vi "LOOP ARM POSITION.vi"(1 "LEFT-RIGHT":string="LEFT", 5 "error in (no error)":errorcluster, 7 "PID Constants ARM":T2={"P Gain"=0.0, "I Gain"=0.0, "D Gain"=0.0, "F Gain"=0.0, "I Zone"=0.0, "Min Output"=-1.0, "Max Output"=1.0} {"Max Output" min=-1.0 max=1.0 step=0.01; "Min Output" min=-1.0 max=1.0 step=0.01; "I Zone" step=0.01; "F Gain" step=0.01; "D Gain" step=0.01; "I Gain" step=0.01; "P Gain" min=0.0 step=0.01}) -> (19 "error out":errorcluster)   [LabVIEW 2020]
uses:
  <vilib>/Rock Robotics/WPI/MotorControl/WPI_MotorControlDeviceRef.ctl
  <vilib>/Rock Robotics/WPI/MotorControl/WPI_MotorControlType.ctl
  <vilib>/Rock Robotics/SystemInterfaces/DIO/FPGA_DIOPWMChannel.ctl
  <vilib>/Rock Robotics/WPI/PWM/WPI_PWMDeadband.ctl
  <vilib>/Rock Robotics/SystemInterfaces/DIO/FPGA_DIOChannel.ctl
  <vilib>/Rock Robotics/WPI/ThirdParty/REV Robotics/REVLib/Typedef/Spark MAX Control Type.ctl
  <vilib>/Rock Robotics/WPI/ThirdParty/REV Robotics/REVLib/Typedef/Spark MAX Limit Direction.ctl
  Robot Global Data.vi
  <vilib>/Rock Robotics/Network Tables/NT Read Number.vi
  <vilib>/Rock Robotics/Network Tables/NT Write Number.vi
panel:
  in  "INPUT STROKE":dbl(slide) min=0.0 max=23.5 scale=0.0..23.5
  in  "INPUT ARM":dbl(slide) min=-3.5 max=4.5 scale=-3.5..4.5
  in  "TESTING?":bool
  out "REV Limit":T1
  out "FWD Limit":T1
  in  "PID Constants Climber":T2={"P Gain"=0.0, "I Gain"=0.0, "D Gain"=0.0, "F Gain"=0.0, "I Zone"=0.0, "Min Output"=-1.0, "Max Output"=1.0} {"Max Output" min=-1.0 max=1.0 step=0.01; "Min Output" min=-1.0 max=1.0 step=0.01; "I Zone" step=0.01; "F Gain" step=0.01; "D Gain" step=0.01; "I Gain" step=0.01; "P Gain" min=0.0 step=0.01}
  out "Position 2":dbl
  out "Output 2":dbl
  out "PID Chart STROKE":T3(graph)
  in  "NT arm string":string="ARM"
  in  "nt set pos string":string="/setPOS"
  out "MotorControlDevRef out":T4={"DeviceStatus"={"status"=FALSE, "code"=0, "source"=""}, "Type"=enum."PWM", "PWM"={"PWM Channel"=enum."Invalid", "DeadBand"={"Name"="", "maxPositivePwm"=0, "minPositivePwm"=0, "centerPwm"=0, "maxNegativePwm"=0, "minNegativePwm"=0, "angularRange"=0}}, "CAN"={"Device Number"=0, "SetOutput VI Ref"=variant, "GetOutput VI Ref"=variant, "Enable VI Ref"=variant, "Disable VI Ref"=variant, "Data"=variant}, "Invert"=FALSE, "DIO PWM"={"PWM \"Enable\" Channel"=enum."Invalid", "DIOChannel"=enum."Invalid", "PWM Rate"=0.0}}
  out "Position":dbl
  out "Output":dbl
  in  "ARM devref in":T4={"DeviceStatus"={"status"=FALSE, "code"=0, "source"=""}, "Type"=enum."PWM", "PWM"={"PWM Channel"=enum."Invalid", "DeadBand"={"Name"="", "maxPositivePwm"=0, "minPositivePwm"=0, "centerPwm"=0, "maxNegativePwm"=0, "minNegativePwm"=0, "angularRange"=0}}, "CAN"={"Device Number"=0, "SetOutput VI Ref"=variant, "GetOutput VI Ref"=variant, "Enable VI Ref"=variant, "Disable VI Ref"=variant, "Data"=variant}, "Invert"=FALSE, "DIO PWM"={"PWM \"Enable\" Channel"=enum."Invalid", "DIOChannel"=enum."Invalid", "PWM Rate"=0.0}}
  out "PID Chart ANGLE":T3(graph)
  # "EXECUTION to SHARED RE-ENTRANT"
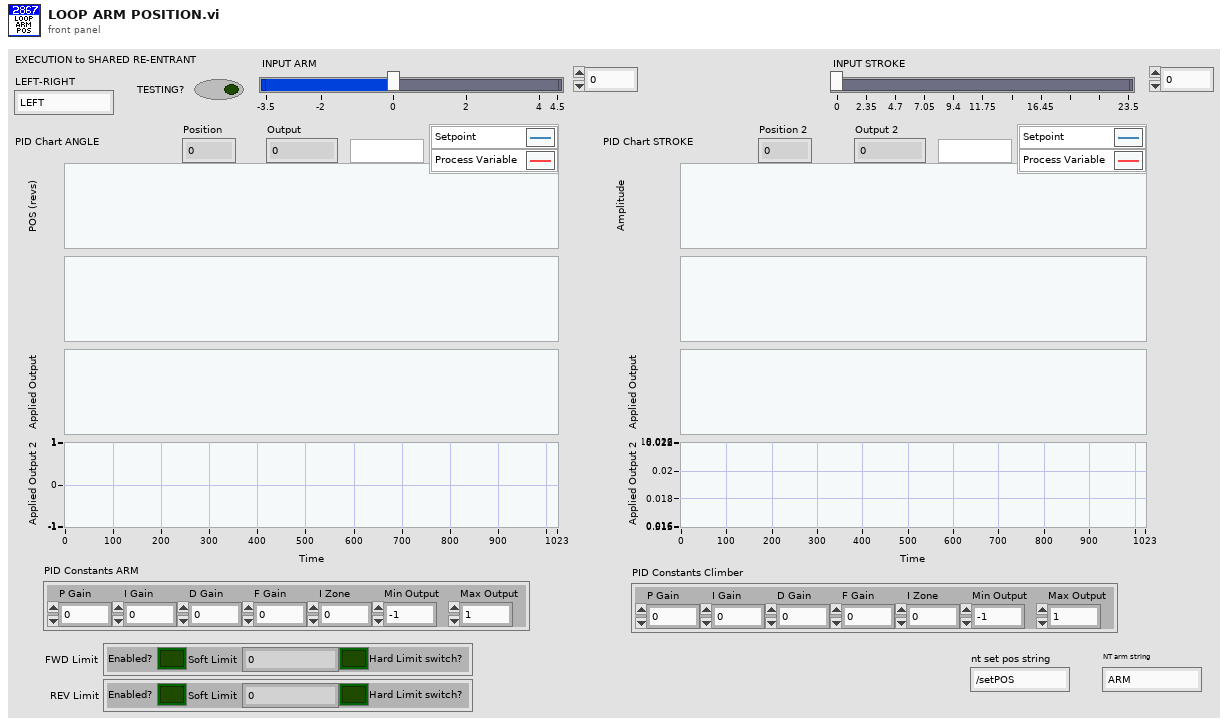
[diagram p1: front panel]
types:
  T1 = cluster{"Enabled?":bool, "Soft Limit":dbl, "Hard Limit switch?":bool}
  T2 = cluster{"P Gain":dbl, "I Gain":dbl, "D Gain":dbl, "F Gain":dbl, "I Zone":dbl, "Min Output":dbl, "Max Output":dbl}
  T3 = cluster{"Sensor Position":dbl, "Sensor Position":dbl, "Setpoint":dbl, "Applied Output":dbl}
  T4 = typedef "WPI_MotorControlDeviceRef.ctl" = cluster{"DeviceStatus":errorcluster, "Type":T5, "PWM":cluster{"PWM Channel":T6, "DeadBand":T7}, "CAN":cluster{"Device Number":u8, "SetOutput VI Ref":variant, "GetOutput VI Ref":variant, "Enable VI Ref":variant, "Disable VI Ref":variant, "Data":variant}, "Invert":bool, "DIO PWM":cluster{"PWM \"Enable\" Channel":T6, "DIOChannel":T8, "PWM Rate":dbl}}
  T5 = typedef "WPI_MotorControlType.ctl" = enum16{"PWM", "CAN", "DIO PWM"}
  T6 = typedef "FPGA_DIOPWMChannel.ctl" = enum8{"PWM 0", "PWM 1", "PWM 2", "PWM 3", "PWM 4", "PWM 5", "PWM 6", "PWM 7", "PWM 8", "PWM 9", "PWM MXP 0", "PWM MXP 1", "PWM MXP 2", "PWM MXP 3", "PWM MXP 4", "PWM MXP 5", "PWM MXP 6", "PWM MXP 7", "PWM MXP 8", "PWM MXP 9", "Invalid"}
  T7 = typedef "WPI_PWMDeadband.ctl" = cluster{"Name":string, "maxPositivePwm":i32, "minPositivePwm":i32, "centerPwm":i32, "maxNegativePwm":i32, "minNegativePwm":i32, "angularRange":u16}
  T8 = typedef "FPGA_DIOChannel.ctl" = enum8{"DIO 0", "DIO 1", "DIO 2", "DIO 3", "DIO 4", "DIO 5", "DIO 6", "DIO 7", "DIO 8", "DIO 9", "DIO MXP 0", "DIO MXP 1", "DIO MXP 2", "DIO MXP 3", "DIO MXP 4", "DIO MXP 5", "DIO MXP 6", "DIO MXP 7", "DIO MXP 8", "DIO MXP 9", "DIO MXP 10", "DIO MXP 11", "DIO MXP 12", "DIO MXP 13", "DIO MXP 14", "DIO MXP 15", "SPI Port CS1", "SPI Port CS2", "SPI Port CS3", "SPI Port MISO", "SPI Port MOSI", "Invalid"}
  T9 = cluster{"MIN":dbl, "MAX":dbl, "convert climber inches to tics":dbl}
  T10 = cluster{"MIN":dbl, "MAX":dbl, "convert arm inches to revs":dbl}
  T11 = typedef "Spark MAX Control Type.ctl" = enum16{"Percent VBus", "Voltage", "Velocity", "Position", "Smart Motion", "Current", "Smart Velocity"}
  T12 = typedef "Spark MAX Limit Direction.ctl" = enum16{"Forward Limit", "Reverse Limit"}
  T13 = cluster{"P Gain":bool, "I Gain":bool, "D Gain":bool, "F Gain":bool, "I Zone":bool, "Min Output":bool, "Max Output":bool}
  T14 = typedef "Spark MAX Status 2 Frame.ctl" = cluster{"Sensor Position":dbl, "IAccum":dbl, "Timestamp":u32}
  T15 = typedef "Spark MAX Status 0 Frame.ctl" = cluster{"Applied Output":dbl, "Faults":T16, "Sticky Faults":T16, "Rsvd":u8, "Status 0 Flags":T17, "Timestamp":u32}
  T16 = typedef "Spark MAX Faults.ctl" = cluster{"Hard Limit Rev":bool, "Hard Limit Fwd":bool, "Soft Limit Fwd":bool, "Soft Limit Rev":bool, "Other Fault":bool, "DRV Fault":bool, "Has Reset?":bool, "CAN RX":bool, "CAN TX":bool, "EEPROM CRC":bool, "Stall":bool, "Sensor Fault":bool, "Motor Type Fault":bool, "IWDT Reset":bool, "Over Current":bool, "Brownout":bool}
  T17 = typedef "Spark MAX Status 0 Flags.ctl" = cluster{"Invert/Brake":bool, "Is Follower":bool}
  T18 = cluster{"Sensor Position":dbl, "Sensor Position":dbl, dbl, "Applied Output":dbl}
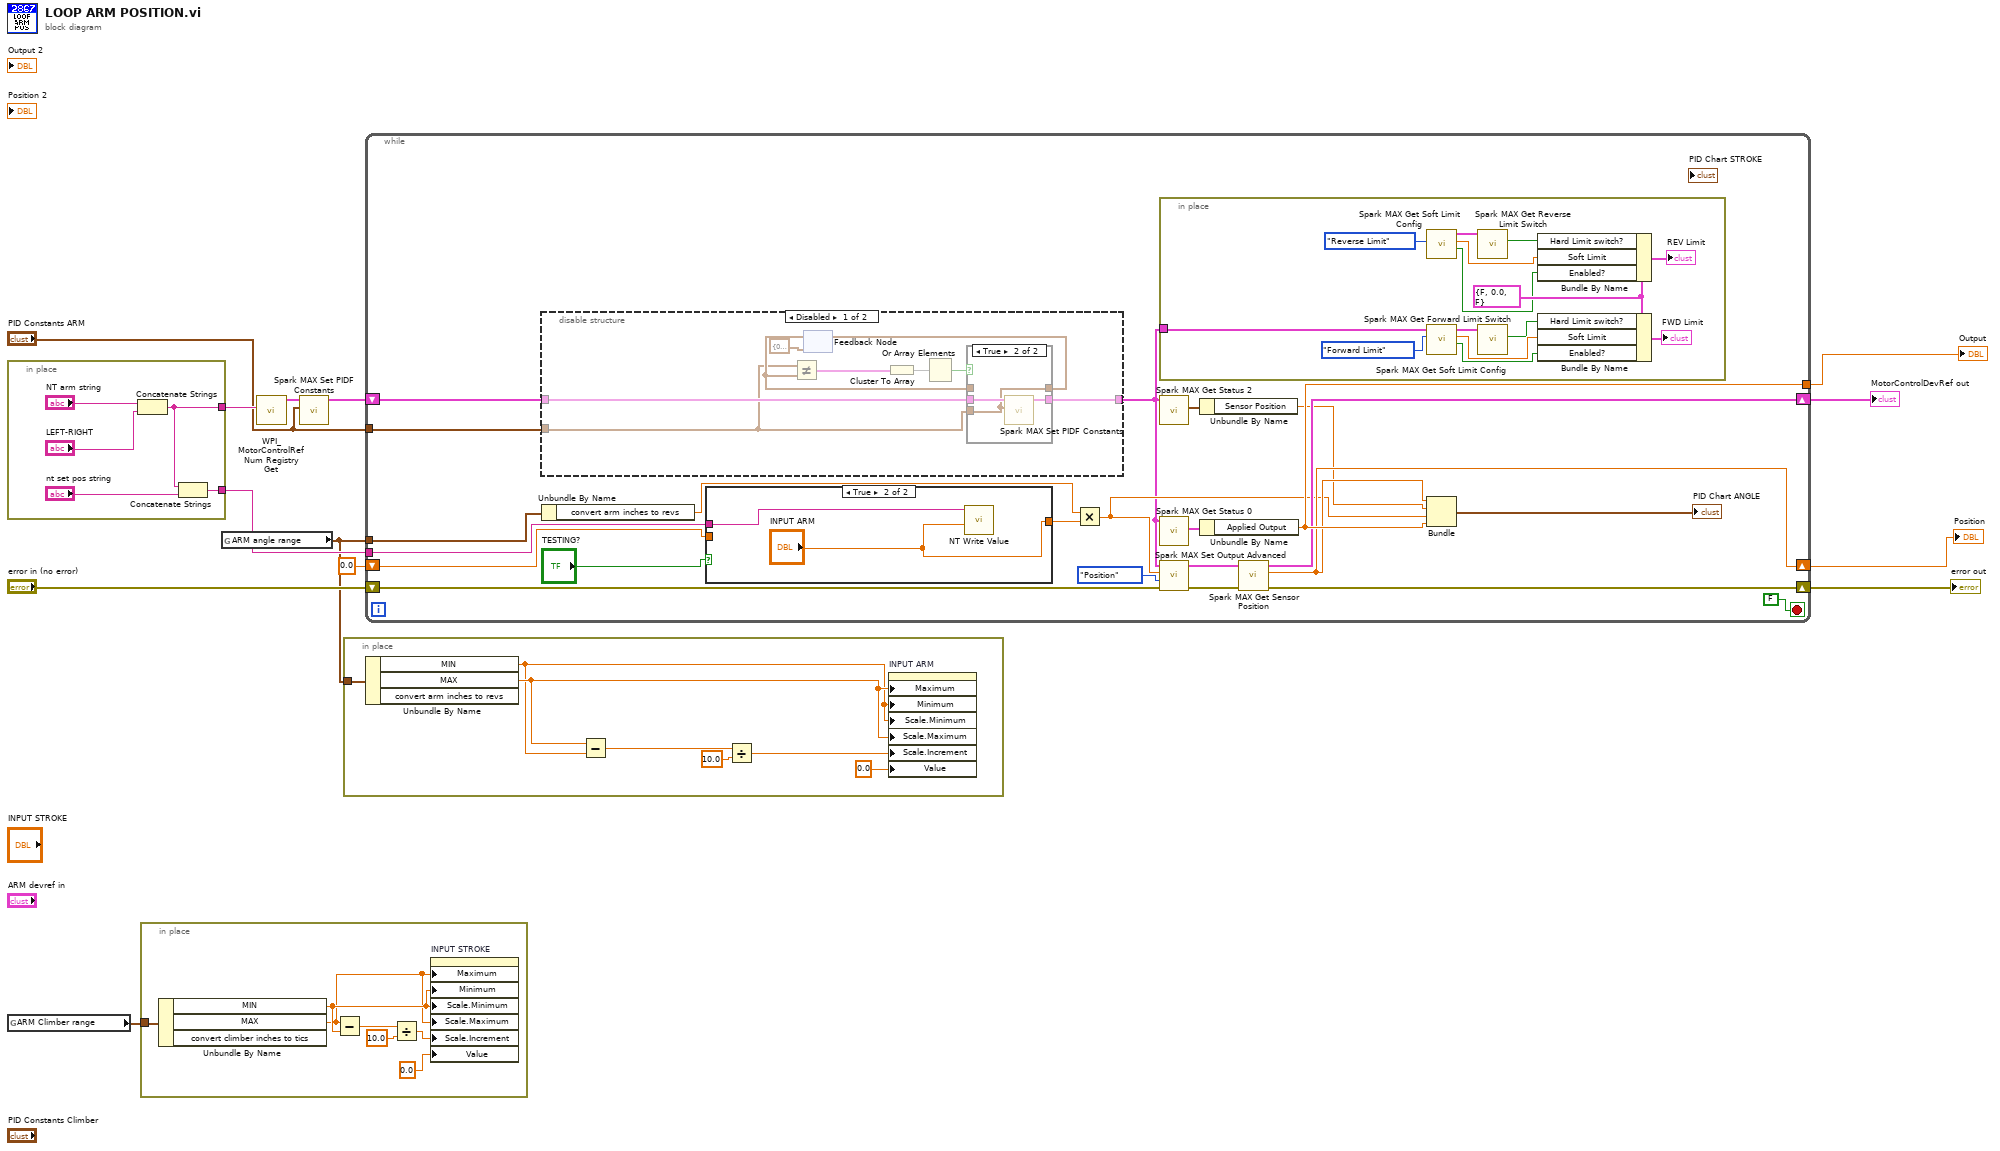
[diagram p0: block diagram]
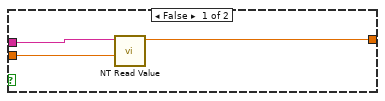
[diagram p4: hidden frame]
diagram:
  n1 = in-place {
    in-place-border: [w15] -> w8
    in-place-border: [w16] -> w4
    n2 = Concatenate Strings("NT arm string", "LEFT-RIGHT") -> (w16:string)
    n3 = Concatenate Strings(w16, "nt set pos string") -> (w15:string)
  }
  n4 = global read "Robot Global Data.vi" "ARM Climber range"() -> (w3:T9)
  n5 = in-place {
    in-place-border: w3 -> [w25]
    n6 = Unbundle By Name(w25) -> ("MIN"=w20:dbl, "MAX"=w19:dbl)  [unwired: 1 out]
    n7 = Subtract(x=w19, y=w20) -> (x-y=w23:dbl)
    n8 = Divide(x=w23, y=10.0) -> (x/y=w21:dbl)
    n9 = property on="INPUT STROKE" class="Slide (strict)"("Maximum"=w19, "Minimum"=w20, "Scale.Minimum"=w20, "Scale.Maximum"=w19, "Scale.Increment"=w21, "Value"=0.0 ("INPUT STROKE")) -> ()  [unwired: 2 in, 2 out]
  }
  n10 = global read "Robot Global Data.vi" "ARM angle range"() -> (w6:T10)
  n11 = call <vilib>:"WPI_MotorControlRefNum Registry Get.vi"("refnum name"=w4) -> ("MotorControlDevRef"=w5:T4)  [unwired: 9 in, 1 out]
  n12 = call <vilib>:"Spark MAX Set PIDF Constants.vi"("PID Constants"="PID Constants ARM", "MotorControlDeviceRef"=w5) -> ("MotorControlDeviceRef"=w2:T4)  [unwired: 8 in, 1 out]
  n13 = in-place {
    in-place-border: w6 -> [w32]
    n14 = Unbundle By Name(w32) -> ("MIN"=w30:dbl, "MAX"=w31:dbl)  [unwired: 1 out]
    n15 = Subtract(x=w31, y=w30) -> (x-y=w29:dbl)
    n16 = Divide(x=w29, y=10.0) -> (x/y=w27:dbl)
    n17 = property on="INPUT ARM" class="Slide (strict)"("Maximum"=w31, "Minimum"=w30, "Scale.Minimum"=w30, "Scale.Maximum"=w31, "Scale.Increment"=w27, "Value"=0.0 ("INPUT ARM")) -> ()  [unwired: 2 in, 2 out]
  }
  n18 = while {
    tunnel: [w54] -> w12
    shift-right: [w55] -> w13
    shift-left: "error in (no error)" -> [w53]
    shift-right: [w50] -> w9
    shift-left: w2 -> [w52]
    shift-right: [w51] -> w10
    shift-left: 0.0 ("ARM Setpoint") -> [w36]
    tunnel: w6 -> [w41]
    tunnel: w8 -> [w40]
    tunnel: "PID Constants ARM" -> [w33]
    stop <- FALSE stop-if-true
    n19 = disable-structure shown="Disabled" {
      disable-tunnel: w52 -> [w64 _]
      disable-tunnel: [w57 _] -> w35
      disable-tunnel: w33 -> [w56 _]
      frame Disabled {
        n20 = feedback #1(T2 {"P Gain"=0.0, "I Gain"=0.0, "D Gain"=0.0, "F Gain"=0.0, "I Zone"=0.0, "Min Output"=0.0, "Max Output"=0.0} ("PID Constants")) -> (w63:T2)
        n21 = Not Equal?(x=w56, y=w63) -> (x != y?=w58:T13)
        n22 = Cluster To Array(cluster=w58) -> (array=w59:bool[])
        n23 = Or Array Elements(Boolean array=w59) -> (logical OR=w61:bool)
        n24 = case shown="True" w61 {
          tunnel: w64 -> [w65 w69]
          tunnel: w56 -> [_ w67]
          tunnel: [w66 w67] -> w62
          tunnel: w63 -> [w66 _]
          tunnel: [w65 w68] -> w57
          frame False {
          }
          frame True {
            n25 = call <vilib>:"Spark MAX Set PIDF Constants.vi"("PID Constants"=w67, "MotorControlDeviceRef"=w69) -> ("MotorControlDeviceRef"=w68:T4)  [unwired: 8 in, 1 out]
          }
        }
        n26 = feedback-in #1(w62) -> ()
      }
      frame Enabled {
      }
    }
    n27 = Unbundle By Name(w41) -> ("convert arm inches to revs"=w38:dbl)
    n28 = case shown="True" "TESTING?" {
      tunnel: w40 -> [w72 w74]
      tunnel: [w71 "INPUT ARM"] -> w39
      tunnel: w36 -> [w70 _]
      frame False {
        n29 = call-poly <vilib>:"NT Read Value.vi"("Default Value"=w70, "Name"=w72) -> ("Numeric"=w71:dbl)  [unwired: 8 in, 1 out]
      }
      frame True {
        n30 = call-poly <vilib>:"NT Write Value.vi"("Numeric"="INPUT ARM", "Name"=w74) -> ()  [unwired: 9 in, 1 out]
      }
    }
    n31 = Multiply(x=w38, y=w39) -> (x*y=w37:dbl)
    n32 = in-place {
      in-place-border: w35 -> [w88]
      w80 = T1 {"Enabled?"=FALSE, "Soft Limit"=0.0, "Hard Limit switch?"=FALSE} ("FWD Limit")
      n33 = call <vilib>:"Spark MAX Get Soft Limit Config.vi"("Soft Limit Switch"=Spark_MAX_Limit_Direction."Reverse Limit") -> ("Enabled?"=w77:bool, "Soft Limit"=w78:dbl, "MotorControlDeviceRef out"=w76:T4)  [unwired: 7 in, 1 out]
      n34 = call <vilib>:"Spark MAX Get Soft Limit Config.vi"("Soft Limit Switch"=Spark_MAX_Limit_Direction."Forward Limit", "MotorControlDeviceRef in"=w88) -> ("Enabled?"=w82:bool, "Soft Limit"=w85:dbl, "MotorControlDeviceRef out"=w86:T4)  [unwired: 6 in, 1 out]
      n35 = call <vilib>:"Spark MAX Get Reverse Limit Switch.vi"("MotorControlDevRef in"=w76) -> ("Hard Limit Rev"=w75:bool)  [unwired: 7 in, 3 out]
      n36 = call <vilib>:"Spark MAX Get Forward Limit Switch.vi"("MotorControlDevRef in"=w86) -> ("Hard Limit Fwd"=w83:bool)  [unwired: 7 in, 3 out]
      n37 = Bundle By Name(cluster=w80, "Hard Limit switch?"=w75, "Soft Limit"=w78, "Enabled?"=w77) -> (→"REV Limit":T1)
      n38 = Bundle By Name(cluster=w80, "Hard Limit switch?"=w83, "Soft Limit"=w85, "Enabled?"=w82) -> (→"FWD Limit":T1)
    }
    n39 = call <vilib>:"Spark MAX Get Status 2.vi"("MotorControlDevRef"=w35) -> ("Stat 2"=w45:T14)  [unwired: 7 in, 3 out]
    n40 = call <vilib>:"Spark MAX Get Status 0.vi"("MotorControlDevRef"=w35) -> ("Status 0"=w49:T15)  [unwired: 7 in, 3 out]
    n41 = call <vilib>:"Spark MAX Set Output Advanced.vi"("error in (no error)"=w53, "Control Mode"=Spark_MAX_Control_Type."Position", "Setpoint"=w37, "MotorControlDevRef"=w35) -> ("error out"=w43:errorcluster, "MotorControlDevRef"=w44:T4)  [unwired: 6 in]
    n42 = Unbundle By Name(w45) -> ("Sensor Position"=w46:dbl)
    n43 = Unbundle By Name(w49) -> ("Applied Output"=w54:dbl)
    n44 = call <vilib>:"Spark MAX Get Sensor Position.vi"("error in (no error)"=w43, "MotorControlDevRef in"=w44) -> ("error out"=w55:errorcluster, "Sensor Position"=w51:dbl, "MotorControlDevRef out"=w50:T4)  [unwired: 6 in, 1 out]
    n45 = Bundle("Sensor Position"=w51, "Sensor Position"=w46, w37, "Applied Output"=w54) -> (→"PID Chart ANGLE":T18)  [unwired: 1 in]
  }
  "Output" <- w12
  "error out" <- w13
  "Position" <- w10
  "MotorControlDevRef out" <- w9
